vi "D_control.vi"(8 "Kd":dbl=500.0 format="%#_13g", 9 "Past Measures":dbl[](array[numeric]), 11 "Feedback error":dbl[](array[numeric])) -> (3 "D control":dbl[](array[numeric]))   [LabVIEW 2021, in "System.lvclass"]
uses:
  System.lvclass
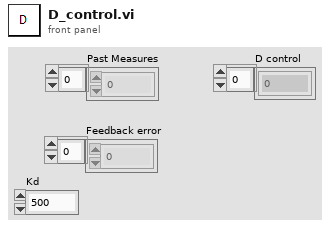
[diagram p1: front panel]
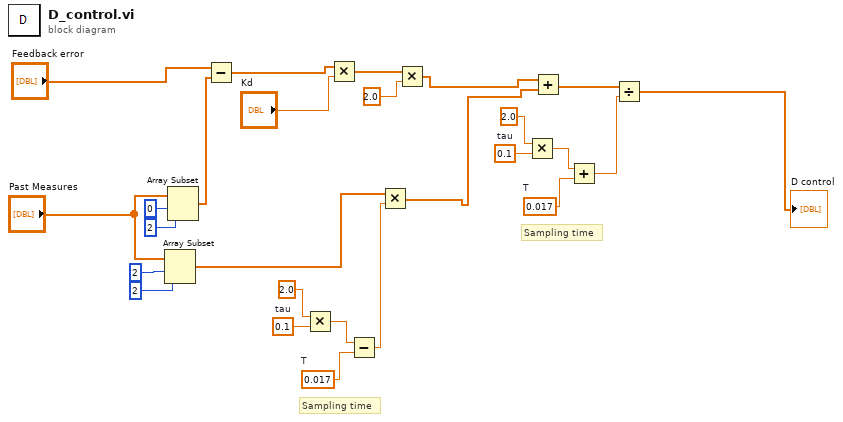
[diagram p0: block diagram]
diagram:
  w5 = 0.1  # tau
  w7 = 0.017  # T
  w12 = 0.1  # tau
  w14 = 0.017  # T
  # "Sampling time"
  # "Sampling time"
  n1 = Array Subset(array="Past Measures", index=2, length=2) -> (w3:dbl[])
  n2 = Array Subset(array="Past Measures", index=0, length=2) -> (w19:dbl[])
  n3 = Subtract(x="Feedback error", y=w19) -> (x-y=w18:dbl[])
  n4 = Multiply(x=2.0, y=w5) -> (x*y=w6:dbl)
  n5 = Multiply(x=w18, y="Kd") -> (x*y=w17:dbl[])
  n6 = Subtract(x=w6, y=w7) -> (x-y=w2:dbl)
  n7 = Multiply(x=w3, y=w2) -> (x*y=w1:dbl[])
  n8 = Multiply(x=w17, y=2.0) -> (x*y=w10:dbl[])
  n9 = Multiply(x=2.0, y=w12) -> (x*y=w13:dbl)
  n10 = Add(x=w10, y=w1) -> (x+y=w9:dbl[])
  n11 = Add(x=w13, y=w14) -> (x+y=w15:dbl)
  n12 = Divide(x=w9, y=w15) -> (x/y=→"D control":dbl[])
